vi "Set PWM Enable.vi"(8 "error in (no error)":errorcluster, 9 "Enable":bool, 10 "Channel":i32, 11 "VISA resource name in":refnum<visa-resource-name>) -> (0 "error out":errorcluster, 3 "VISA resource name":refnum<visa-resource-name>)   [LabVIEW 2020, in "CTI-Visa.lvlib"]
uses:
  CTI-Visa.lvlib
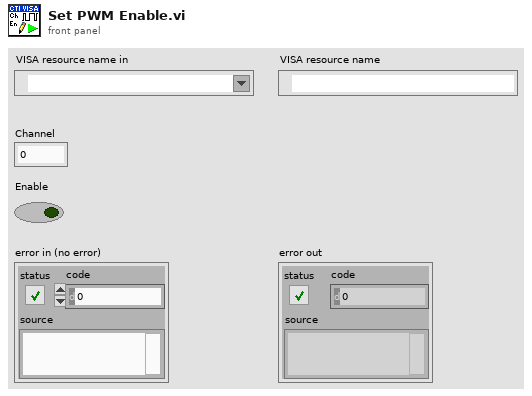
[diagram p1: front panel]
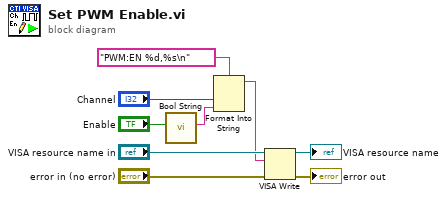
[diagram p0: block diagram]
diagram:
  n1 = call "Bool String.vi"("Bool"="Enable") -> ("String"=w6:string)  [unwired: 10 in]
  n2 = Format Into String(format string="PWM:EN %d,%s\n", "Channel", w6) -> (resulting string=w4:string)  [unwired: 2 in, 1 out]
  n3 = VISA Write(VISA resource name="VISA resource name in", write buffer=w4, error in (no error)="error in (no error)") -> (VISA resource name out=→"VISA resource name":refnum<visa-resource-name>, error out=→"error out":errorcluster)  [unwired: 1 out]
